vi "例程40-Butterworth滤波器.vi"() -> ()   [LabVIEW 2016]
uses:
  <vilib>/Analysis/3filter.llb/Filter Passband Type.ctl
  <vilib>/Analysis/3filter.llb/Butterworth Filter (DBL).vi
  <vilib>/Analysis/NI_AALBase.lvlib
panel:
  in  "order":i32=2 caption="阶数"
  out "滤波后波形":dynamicdata(graph)=[{"t0"=timestamp(3624840152.178216 s since 1904-01-01), "dt"=1.0, "Y"=[0.008313893041455774, 0.027077564749554847, 0.052603057730961154, 0.09965386953412836, 0.18542060979120947, 0.3127536552504783, 0.45360469830570405, 0.5705854240861766, 0.6537894327142272, 0.6996815489244336, 0.7131244044360393, 0.6992932875019561, 0.6569350857688493, 0.606194274243568, 0.5567338131797164, 0.4918072218021837, 0.40107320892499154, 0.2800028995036625, 0.1300602297833893, -0.02297645069248578, -0.1607111176455457, -0.2935804442457325, -0.420729622053723, -0.5307632369274562, -0.6157867372474728, -0.6448453577434422, -0.6067923153642607, -0.5364088005351666, -0.4310172519551121, -0.26776928390961685, -0.06045514897741217, 0.17554756519756642, 0.4132799858552561, 0.6102500440075497, 0.7381945705771109, 0.8042014114411505, 0.8298389256079102, 0.8156616164654762, 0.7575984743118653, 0.6358994722042802, 0.4511488759404426, 0.24370430210155475, 0.02579299385794078, -0.21435366635985087, -0.45413033194890834, -0.6444610216219727, -0.77849962931636, -0.8879331261656312, -0.9663514878467536, -0.976447611637649, -0.9097814390529204, -0.7867533271474213, -0.6190120417722595, -0.42060016131435174, -0.23114715422514376, -0.056618395959606875, 0.13829353620888055, 0.3588287324309743, 0.5782784854821433, 0.7560825631461408, 0.8645955488076623, 0.9252210307571977, 0.9353350884748457, 0.8720068192802806, 0.7559633971850531, 0.5916057359546795, 0.3733309584702501, 0.1191097834370623, -0.14098775032036587, -0.36314396232087015, -0.5207810723324197, -0.6288146105673881, -0.7013921335028301, -0.7308103068962257, -0.7266359816873192, -0.699235025722436, -0.6388880440859603, -0.5421269364896684, -0.42133617267822454, -0.2737284923429645, -0.09200041464951916, 0.09729795828232864, 0.2814035736318812, 0.4631466061963897, 0.6282705578572567, 0.7669426039476686, 0.8652693504478073, 0.893347072003901, 0.8293304814204817, 0.6872958524113236, 0.49781821172204815, 0.27591261305956305, 0.027814807137247474, -0.22599465698778004, -0.4547417632279996, -0.6330996953543694, -0.7522466799495424, -0.8324490990505831, -0.8862159521441599, -0.9017710063370687]}]
  out "滤波前波形":dynamicdata(graph)=[{"t0"=timestamp(40.5 s since 1904-01-01), "dt"=0.001, "Y"=[0.4139691136365718, -0.12589317478981388, 0.6178965382659446, 0.628144613809243, 1.2924234313589036, 1.1300004368871035, 0.645596300256186, 0.7199801085636269, 0.6039998063854695, 0.3151834515354206, 0.7681720268535817, -0.11700550371427615, 0.5955827593795073, 0.3797574635795708, 0.22730249428909322, -0.26078796185846315, -0.18297062189626778, -0.8998232598198852, -0.4970687478379508, -0.41753080808087173, -0.7307775810194214, -0.9811650384061817, -0.5691724694693532, -0.98181092120041, -0.3099224858305206, 0.4067890099726897, -0.2603112049638225, -0.02397168972352426, 1.162663020269081, 0.7374703884103352, 1.4007614669219208, 1.3498736922214056, 0.9023409109247756, 0.7143287331496275, 0.19053993456477125, 1.0581720562008492, 0.0785831117137924, 0.5793741458903496, -0.41304632546985065, -0.9283638318967535, -0.49942062877930793, -0.6974617474804558, -1.3565453343487608, -1.4848853879437527, -0.801211322149524, -0.549105299726681, -1.2744242191592607, -1.1845555833655885, -0.3181393734953737, -0.04303393270221359, 0.1403032516973263, 0.12022436641762937, 0.8956475206423922, 0.13511806753219835, 0.24886802590867962, 1.082691488748995, 1.4909357340446645, 1.2451908775236924, 1.338265020629287, 0.23668339043008213, 0.9377478705495048, 0.8995902549558275, -0.4684828735691452, 0.30245906807483885, -0.404140011728105, -0.9483116629511097, -0.9525759193600548, -1.3410198404490086, -0.7214217666475622, -0.5357143427537951, -0.4144236924675174, -1.0637604445328497, -0.1371333667910022, -0.6146199411619193, -0.4095644606440707, -0.24173914427669957, 0.22589191132876763, 0.12522729130719162, 0.27959975375904017, 1.1225882923616295, 0.7152238081572752, 0.7012034641068521, 1.3934886699758295, 0.8075502117666414, 1.2620570951694594, 0.8130938359071335, 0.6470377510213048, -0.38804541662040987, -0.38174861407408917, -0.5590521825674046, -0.6497198779807354, -1.1485917927146827, -1.216407370215231, -1.0222588561590082, -0.9276631811464281, -0.5173439714731591, -0.8069029038196724, -1.066416751370128, -0.5060220399143524, -0.5239115570701325], "attributes"=variant("NI_ChannelName"=variant(string "正弦 ＋均匀噪声"), "NI_ExpIsRelativeTime"=variant(bool TRUE), "NI_ExpStartTimeStamp"=variant(timestamp timestamp(3624840111.5389137 s since 1904-01-01)), "NI_ExpTimeStamp"=variant(timestamp timestamp(3624840152.0389137 s since 1904-01-01)), "NI_ExpXDimension"=variant(string "t"))}]
  in  "停止":bool
  in  "噪声幅值":dbl=0.6
  in  "Amplitude":dbl=1.0 caption="幅值"
  in  "Frequency":dbl=40.0 caption="频率"
  in  "Offset":dbl caption="偏移量"
  in  "filter type":T1 caption="滤波器类型"
  in  "low cutoff freq: fl":dbl=10.0 caption="低截止频率:fl" format="%0.4f"
  in  "high cutoff freq: fh":dbl=10.0 caption="高截止频率:fh" format="%0.2f"
  in  "sampling freq: fs":dbl=200.0 caption="采样频率:fs" format="%0.2f"
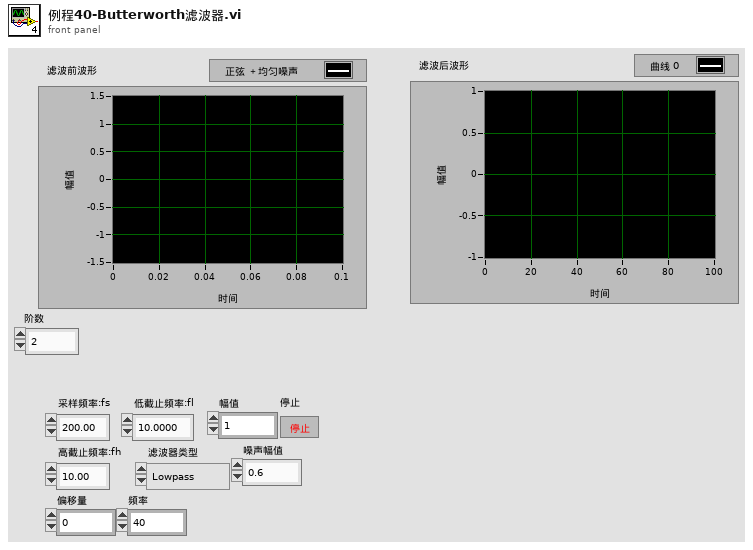
[diagram p1: front panel]
types:
  T1 = typedef "NI_AALBase.lvlib/Filter Passband Type.ctl" = enum32{"Lowpass", "Highpass", "Bandpass", "Bandstop"}
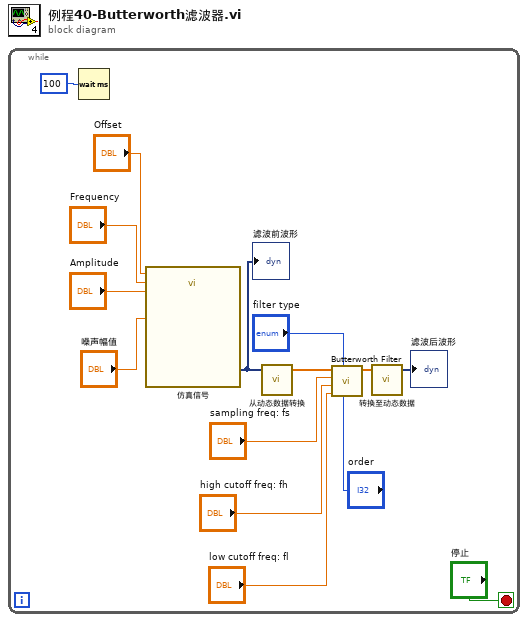
[diagram p0: block diagram]
diagram:
  n1 = while {
    stop <- "停止" stop-if-true
    n2 = Wait (ms)(milliseconds to wait=u32 100 ("等待时间（毫秒）")) -> ()  [unwired: 1 out]
    n3 = call "仿真信号"("Offset"="Offset", "Frequency"="Frequency", "Amplitude"="Amplitude", "噪声幅值"="噪声幅值") -> ("正弦与均匀噪声"=w2:dynamicdata)  [unwired: 10 in, 1 out]
    "滤波前波形" <- w2
    n4 = call "从动态数据转换"("Dynamic Data Type"=w2) -> ("Array"=w15:dbl[])  [unwired: 3 in]
    n5 = call-poly <vilib>:"Butterworth Filter.vi"("order"="order", "filter type"="filter type", "low cutoff freq: fl"="low cutoff freq: fl", "high cutoff freq: fh"="high cutoff freq: fh", "sampling freq: fs"="sampling freq: fs", "X"=w15) -> ("Filtered X"=w4:dbl[])  [unwired: 2 in, 1 out]
    n6 = call "转换至动态数据"("Array"=w4) -> ("Dynamic Data Type"=→"滤波后波形":dynamicdata)  [unwired: 3 in]
  }
